vi "Set_Data.vi"(8 "error in (no error)":errorcluster caption="entrée d'erreur (pas d'erreur)", 11 "Firebase Benches en entrée":refnum<class "Firebase Benches.lvclass">) -> (0 "error out":errorcluster caption="sortie d'erreur", 3 "Firebase Benches en sortie":refnum<class "Firebase Benches.lvclass">)   [LabVIEW 2020, in "Library Instrument & Equipement.lvlib" / "Library FireBase.lvlib" / "Firebase Benches.lvclass"]
doc: "Create New document\nPlease initialise the following values\n - Name BDD\n - Document\n - API Key"
uses:
  Firebase Benches.lvclass
  C:/Users/ngarcin/OneDrive - Altyor/Standard TB/Class/Firebase/Source/Firebase Altyor/Firebase Altyor.lvclass
  C:/Users/ngarcin/OneDrive - Altyor/Standard TB/Class/Firebase/Source/Firebase Driver/Firebase Driver.lvclass
  Firebase Benches.lvclass/Firebase Benches.ctl
  Firebase Altyor/Firebase Altyor.lvclass
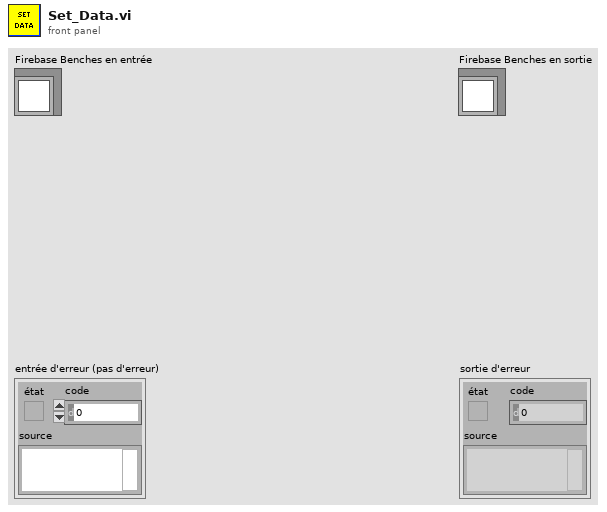
[diagram p1: front panel]
types:
  T1 = cluster{"Result":cluster{"booleanValue":bool}, "CreationDate":cluster{"timestampValue":string}, "Batch":cluster{"stringValue":string}, "SerialNumber":cluster{"stringValue":string}, "EndOfProduction":cluster{"timestampValue":string}, "FW_Version":cluster{"mapValue":cluster{"fields":cluster{"Bootloader":cluster{"mapValue":cluster{"fields":cluster{"File_Name":cluster{"stringValue":string}, "Version":cluster{"mapValue":cluster{"fields":cluster{"Major":cluster{"stringValue":string}, "Minor":cluster{"stringValue":string}}}}, "Checksum":cluster{"stringValue":string}}}}, "SoftDevice":cluster{"mapValue":cluster{"fields":cluster{"File_Name":cluster{"stringValue":string}, "Version":cluster{"mapValue":cluster{"fields":cluster{"Major":cluster{"stringValue":string}, "Minor":cluster{"stringValue":string}}}}, "Checksum":cluster{"stringValue":string}}}}, "DFU":cluster{"mapValue":cluster{"fields":cluster{"File_Name":cluster{"stringValue":string}, "Version":cluster{"mapValue":cluster{"fields":cluster{"Major":cluster{"stringValue":string}, "Minor":cluster{"stringValue":string}}}}, "Checksum":cluster{"stringValue":string}}}}}}}, "PartNumber":cluster{"stringValue":string}, "OrderNumber":cluster{"stringValue":string}, "Operator":cluster{"stringValue":string}}
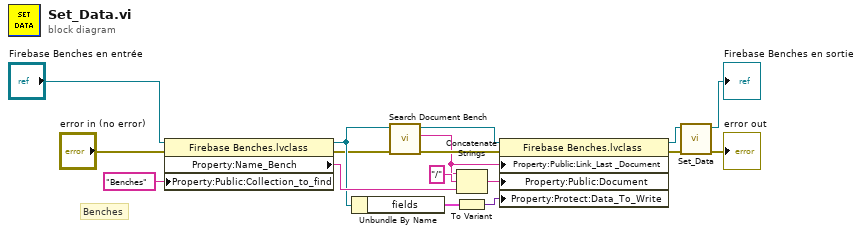
[diagram p0: block diagram]
diagram:
  # "Benches"
  n1 = property class="Firebase Benches.lvclass"(reference="Firebase Benches en entrée", error in="error in (no error)", "Property:Public:Collection_to_find"="Benches" ("Collection_to_find")) -> (reference out=w3:refnum<class "Firebase Benches.lvclass">, error out=w2:errorcluster, "Property:Name_Bench"=w5:string)
  n2 = Unbundle By Name(w3) -> ("fields"=w13:T1)
  n3 = call "Search Document Bench.vi"("entrée d'erreur (pas d'erreur)"=w2, "Firebase Altyor en entrée"=w3) -> ("sortie d'erreur"=w10:errorcluster, "Source"=w7:string, "Firebase Altyor en sortie"=w9:refnum<class "Firebase Benches.lvclass">)  [unwired: 7 in]
  n4 = Concatenate Strings(w7, "/" ("chaîne"), w5) -> (w8:string)
  n5 = To Variant(anything=w13) -> (Variant=w12:variant)
  n6 = property class="Firebase Benches.lvclass"(reference=w9, error in=w10, "Property:Public:Link_Last _Document"=w7, "Property:Public:Document"=w8, "Property:Protect:Data_To_Write"=w12) -> (reference out=w15:refnum<class "Firebase Benches.lvclass">, error out=w14:errorcluster)
  n7 = call-parent "Set_Data.vi"("error in (no error)"=w14, "Firebase Altyor en entrée"=w15) -> ("error out"=→"error out":errorcluster, "Firebase Altyor en sortie"=→"Firebase Benches en sortie":refnum<class "Firebase Benches.lvclass">)  [unwired: 8 in]
